vi "Start of Block (SubVI).vi"(10 "Row #":u16, 11 "Col #":u16) -> (3 "Start?":bool)   [LabVIEW 2015]
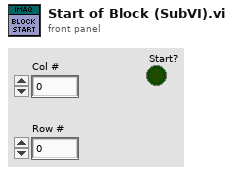
[diagram p1: front panel]
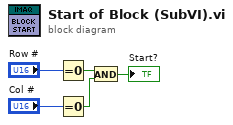
[diagram p0: block diagram]
diagram:
  n1 = Equal To 0?(x="Row #") -> (x = 0?=w1:bool)
  n2 = Equal To 0?(x="Col #") -> (x = 0?=w4:bool)
  n3 = And(x=w1, y=w4) -> (x .and. y?=→"Start?":bool)
